vi "Set Bus.vi"(8 "error in (no error)":errorcluster, 10 "Bus":refnum<class "Local Bus.lvclass">, 11 "Local Bus_Int in":refnum<class "Local Bus_Int.lvclass">) -> (0 "error out":errorcluster, 3 "Local Bus_Int out":refnum<class "Local Bus_Int.lvclass">)   [LabVIEW 2021, in "Local Bus_Int.lvclass"]
uses:
  Local Bus_Int.lvclass
  Local Bus.lvclass
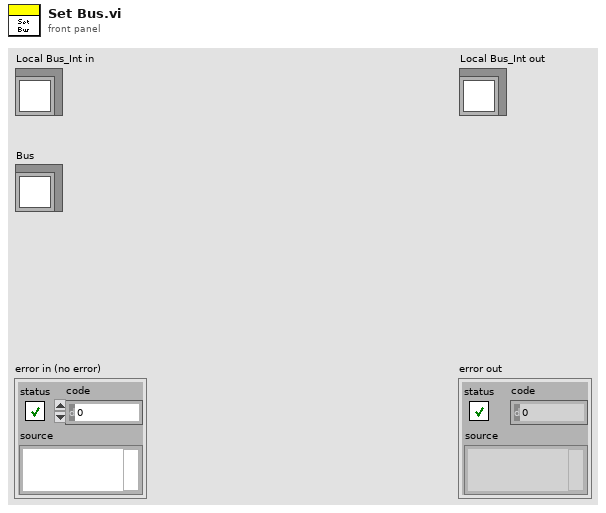
[diagram p1: front panel]
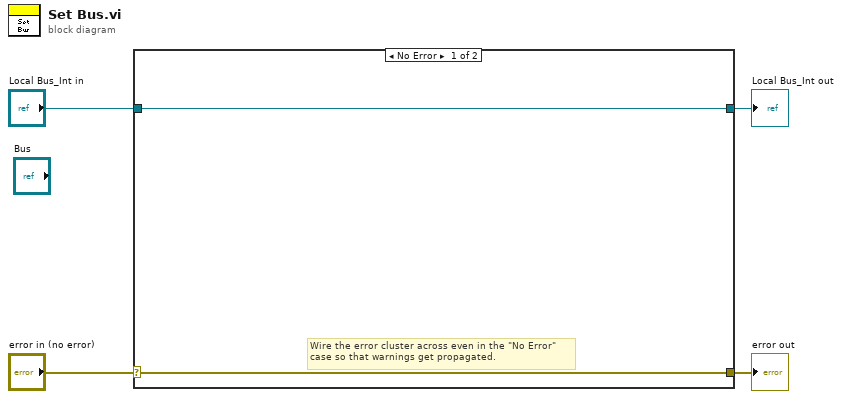
[diagram p0: block diagram]
diagram:
  n1 = case shown="No Error" "error in (no error)" {
    selector: "error in (no error)" -> [w5 w8]
    tunnel: [w5 w8] -> w3
    tunnel: [w6 w7] -> w1
    tunnel: "Local Bus_Int in" -> [w6 w7]
    frame No Error {
      # "Wire the error cluster across even in the \"No Error\"\ncase so that warnings get propagated."
    }
    frame Error {
    }
  }
  "error out" <- w3
  "Local Bus_Int out" <- w1
